vi "fpga_1DAC_sine_and_1ADC_W_risingedge_R_trailingedge_stacked.vi"() -> ()   [LabVIEW 2018]
uses:
  <vilib>/eio/EIONode/EIONode.xnode
  <vilib>/rvi/eio/common/nirviEmuTemplateMethod_errors.vi
panel:
  in  "delay 4 (us)":u32=350
  in  "delay3 (us)":u32=350
  in  "delay 2 (us)":u32=350
  in  "delay 1 (us)":u32=350
  out "ADC4 read":bool[](array[boolean])
  in  "ADC1 write":bool[](array[boolean])=[FALSE, FALSE, FALSE, FALSE, FALSE, TRUE, FALSE, FALSE, FALSE, FALSE, FALSE, FALSE, FALSE, FALSE, FALSE, FALSE]
  out "ADC3 read":bool[](array[boolean])
  in  "ADC4 write":bool[](array[boolean])=[FALSE, FALSE, TRUE, TRUE, FALSE, TRUE, FALSE, FALSE, FALSE, FALSE, FALSE, FALSE, FALSE, FALSE, FALSE, FALSE]
  in  "ADC3 write":bool[](array[boolean])=[FALSE, FALSE, TRUE, FALSE, FALSE, TRUE, FALSE, FALSE, FALSE, FALSE, FALSE, FALSE, FALSE, FALSE, FALSE, FALSE]
  out "ADC2 read":bool[](array[boolean])
  in  "DAC 1 write":bool[](array[boolean])=[FALSE, FALSE, FALSE, FALSE, FALSE, FALSE, FALSE, FALSE, FALSE, FALSE, FALSE, FALSE, FALSE, FALSE, FALSE, FALSE]
  out "ADC1 read":bool[](array[boolean])
  in  "ADC2 write":bool[](array[boolean])=[FALSE, FALSE, FALSE, TRUE, FALSE, TRUE, FALSE, FALSE, FALSE, FALSE, FALSE, FALSE, FALSE, FALSE, FALSE, FALSE]
  in  "delay (us)":u32=350
  in  "Stop":bool
  in  "DAC 2 write":bool[](array[boolean])=[FALSE, FALSE, FALSE, FALSE, FALSE, FALSE, FALSE, FALSE, FALSE, FALSE, FALSE, FALSE, FALSE, FALSE, FALSE, FALSE]
  in  "DAC 3 write":bool[](array[boolean])=[FALSE, FALSE, FALSE, FALSE, FALSE, FALSE, FALSE, FALSE, FALSE, FALSE, FALSE, FALSE, FALSE, FALSE, FALSE, FALSE]
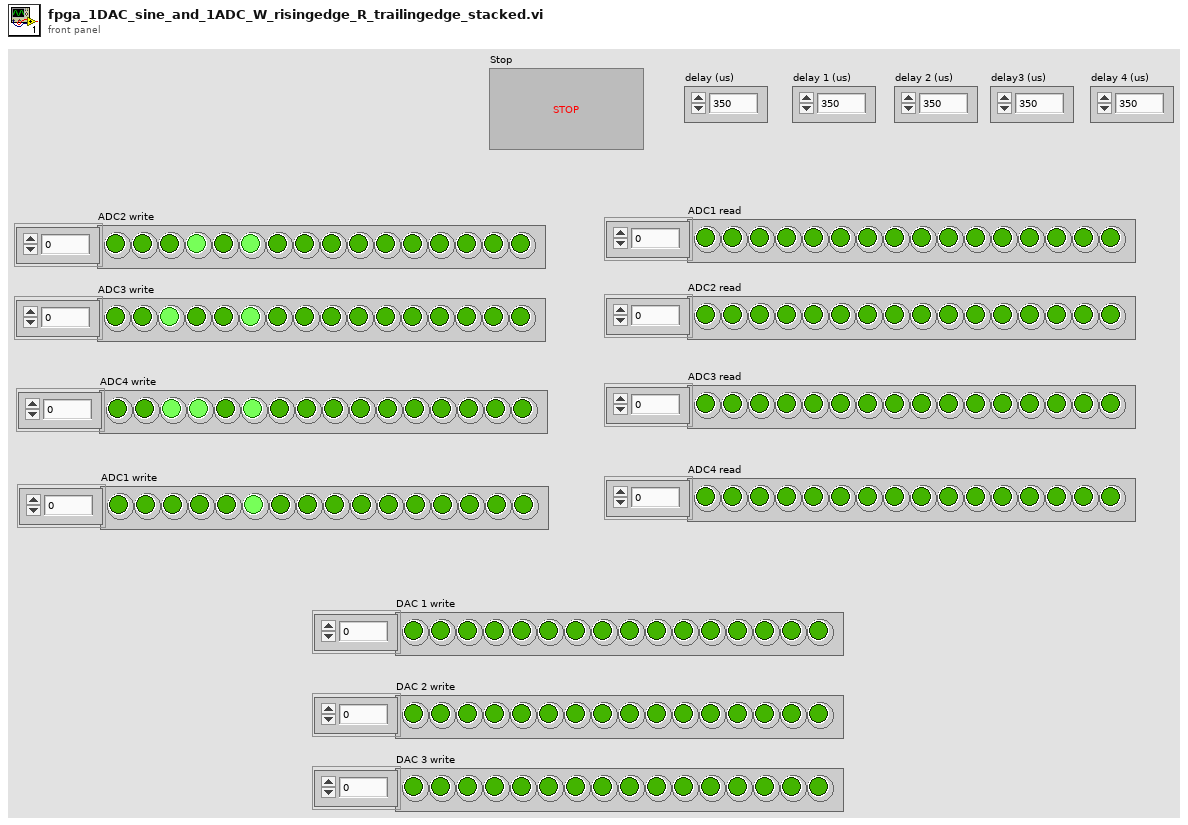
[diagram p1: front panel]
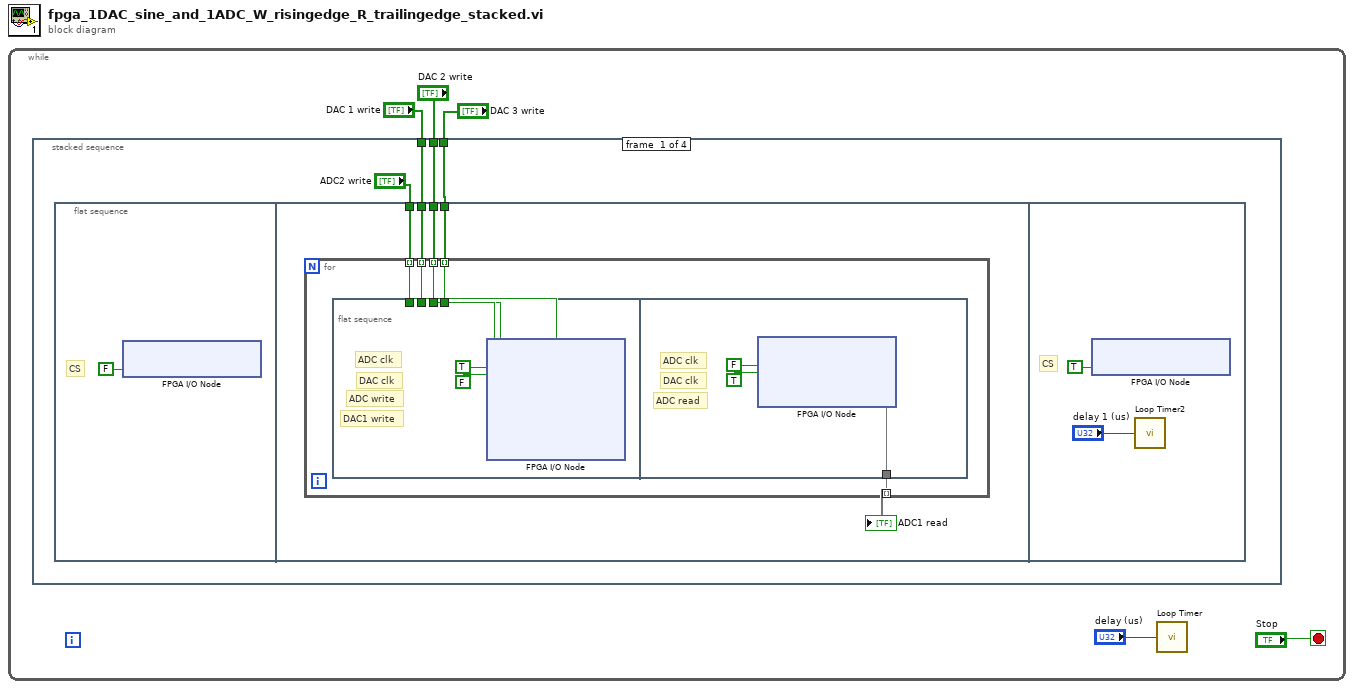
[diagram p0: block diagram]
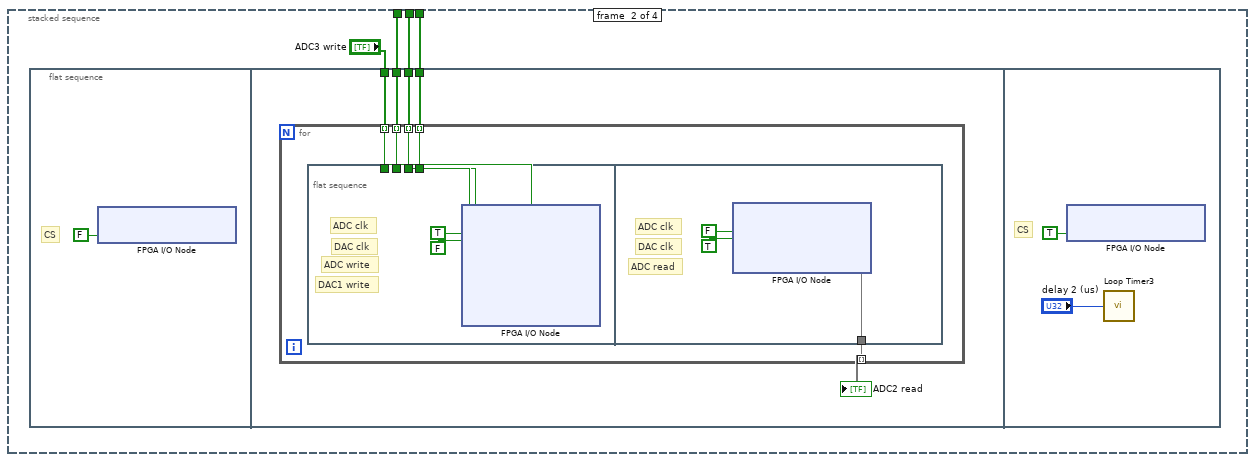
[diagram p2: hidden frame]
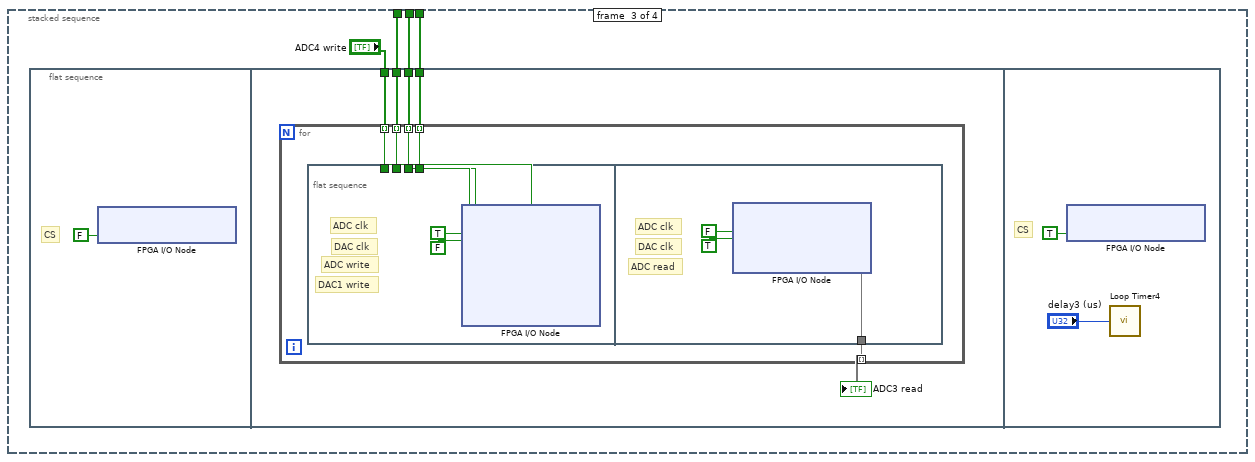
[diagram p3: hidden frame]
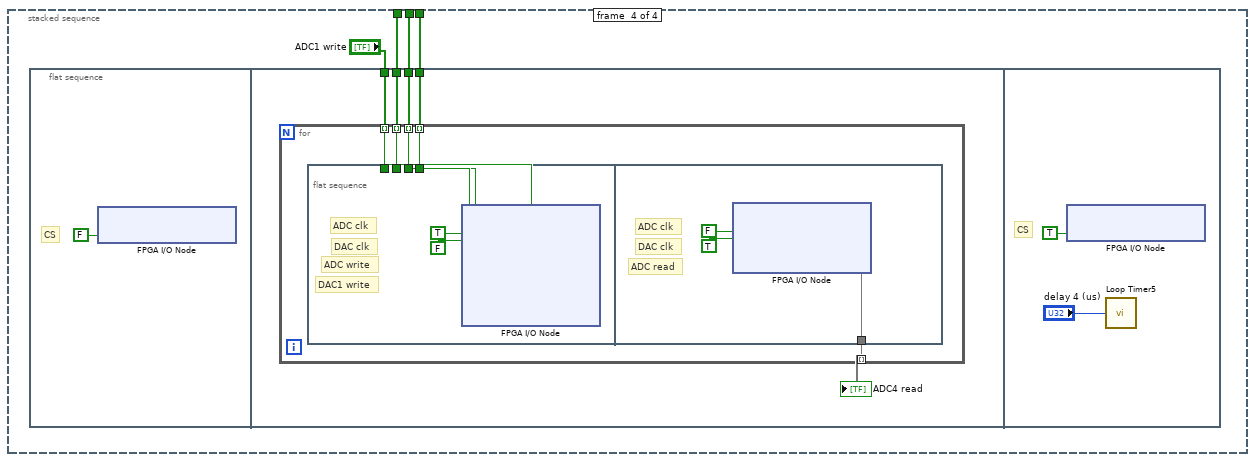
[diagram p4: hidden frame]
diagram:
  n1 = while {
    stop <- "Stop" stop-if-true
    n2 = stacked-sequence {
      tunnel: "DAC 3 write" -> [w8 w32 w58 w84]
      tunnel: "DAC 2 write" -> [w7 w33 w59 w85]
      tunnel: "DAC 1 write" -> [w6 w34 w60 w86]
      frame #0 {
        n3 = flat-sequence {
          tunnel: w6 -> [w15]
          tunnel: "ADC2 write" -> [w14]
          tunnel: w7 -> [w12]
          tunnel: w8 -> [w11]
          frame #0 {
            # "CS"
            n4 = xnode "FPGA I/O Node"("ConnectorA/DIO4"=FALSE) -> ()  [unwired: 1 in, 1 out]
          }
          frame #1 {
            n5 = for {
              tunnel: w15 -> [w20] mode=indexing
              tunnel: w14 -> [w19] mode=indexing
              tunnel: [w18] -> w13 mode=indexing
              tunnel: w12 -> [w17] mode=indexing
              tunnel: w11 -> [w16] mode=indexing
              n6 = flat-sequence {
                tunnel: w20 -> [w23]
                tunnel: w19 -> [w24]
                tunnel: w17 -> [w22]
                tunnel: w16 -> [w21]
                tunnel: [w27] -> w18
                frame #0 {
                  # "DAC1 write"
                  # "ADC write"
                  # "DAC clk"
                  # "ADC clk"
                  n7 = xnode "FPGA I/O Node"("ConnectorA/DIO3"=TRUE, "ConnectorA/DIO5"=FALSE, "ConnectorA/DIO2"=w24, "ConnectorA/DIO6"=w23, "ConnectorA/DIO7"=w22, "ConnectorA/DIO8"=w21) -> ()  [unwired: 6 in, 6 out]
                }
                frame #1 {
                  # "ADC read"
                  # "DAC clk"
                  # "ADC clk"
                  n8 = xnode "FPGA I/O Node"("ConnectorA/DIO3"=FALSE, "ConnectorA/DIO5"=TRUE) -> ("ConnectorA/DIO1"=w27)  [unwired: 3 in, 3 out]
                }
              }
            }
            "ADC1 read" <- w13
          }
          frame #2 {
            # "CS"
            n9 = xnode "FPGA I/O Node"("ConnectorA/DIO4"=TRUE) -> ()  [unwired: 1 in, 1 out]
            n10 = call "Loop Timer2"("Count(Ticks)"="delay 1 (us)") -> ()  [unwired: 1 out]
          }
        }
      }
      frame #1 {
        n11 = flat-sequence {
          tunnel: w34 -> [w41]
          tunnel: "ADC3 write" -> [w40]
          tunnel: w33 -> [w38]
          tunnel: w32 -> [w37]
          frame #0 {
            # "CS"
            n12 = xnode "FPGA I/O Node"("ConnectorA/DIO4"=FALSE) -> ()  [unwired: 1 in, 1 out]
          }
          frame #1 {
            n13 = for {
              tunnel: w41 -> [w46] mode=indexing
              tunnel: w40 -> [w45] mode=indexing
              tunnel: [w44] -> w39 mode=indexing
              tunnel: w38 -> [w43] mode=indexing
              tunnel: w37 -> [w42] mode=indexing
              n14 = flat-sequence {
                tunnel: w46 -> [w49]
                tunnel: w45 -> [w50]
                tunnel: w43 -> [w48]
                tunnel: w42 -> [w47]
                tunnel: [w53] -> w44
                frame #0 {
                  # "DAC1 write"
                  # "ADC write"
                  # "DAC clk"
                  # "ADC clk"
                  n15 = xnode "FPGA I/O Node"("ConnectorA/DIO3"=TRUE, "ConnectorA/DIO5"=FALSE, "ConnectorA/DIO2"=w50, "ConnectorA/DIO6"=w49, "ConnectorA/DIO7"=w48, "ConnectorA/DIO8"=w47) -> ()  [unwired: 6 in, 6 out]
                }
                frame #1 {
                  # "ADC read"
                  # "DAC clk"
                  # "ADC clk"
                  n16 = xnode "FPGA I/O Node"("ConnectorA/DIO3"=FALSE, "ConnectorA/DIO5"=TRUE) -> ("ConnectorA/DIO1"=w53)  [unwired: 3 in, 3 out]
                }
              }
            }
            "ADC2 read" <- w39
          }
          frame #2 {
            # "CS"
            n17 = xnode "FPGA I/O Node"("ConnectorA/DIO4"=TRUE) -> ()  [unwired: 1 in, 1 out]
            n18 = call "Loop Timer3"("Count(Ticks)"="delay 2 (us)") -> ()  [unwired: 1 out]
          }
        }
      }
      frame #2 {
        n19 = flat-sequence {
          tunnel: w60 -> [w67]
          tunnel: "ADC4 write" -> [w66]
          tunnel: w59 -> [w64]
          tunnel: w58 -> [w63]
          frame #0 {
            # "CS"
            n20 = xnode "FPGA I/O Node"("ConnectorA/DIO4"=FALSE) -> ()  [unwired: 1 in, 1 out]
          }
          frame #1 {
            n21 = for {
              tunnel: w67 -> [w72] mode=indexing
              tunnel: w66 -> [w71] mode=indexing
              tunnel: [w70] -> w65 mode=indexing
              tunnel: w64 -> [w69] mode=indexing
              tunnel: w63 -> [w68] mode=indexing
              n22 = flat-sequence {
                tunnel: w72 -> [w75]
                tunnel: w71 -> [w76]
                tunnel: w69 -> [w74]
                tunnel: w68 -> [w73]
                tunnel: [w79] -> w70
                frame #0 {
                  # "DAC1 write"
                  # "ADC write"
                  # "DAC clk"
                  # "ADC clk"
                  n23 = xnode "FPGA I/O Node"("ConnectorA/DIO3"=TRUE, "ConnectorA/DIO5"=FALSE, "ConnectorA/DIO2"=w76, "ConnectorA/DIO6"=w75, "ConnectorA/DIO7"=w74, "ConnectorA/DIO8"=w73) -> ()  [unwired: 6 in, 6 out]
                }
                frame #1 {
                  # "ADC read"
                  # "DAC clk"
                  # "ADC clk"
                  n24 = xnode "FPGA I/O Node"("ConnectorA/DIO3"=FALSE, "ConnectorA/DIO5"=TRUE) -> ("ConnectorA/DIO1"=w79)  [unwired: 3 in, 3 out]
                }
              }
            }
            "ADC3 read" <- w65
          }
          frame #2 {
            # "CS"
            n25 = xnode "FPGA I/O Node"("ConnectorA/DIO4"=TRUE) -> ()  [unwired: 1 in, 1 out]
            n26 = call "Loop Timer4"("Count(Ticks)"="delay3 (us)") -> ()  [unwired: 1 out]
          }
        }
      }
      frame #3 {
        n27 = flat-sequence {
          tunnel: w86 -> [w93]
          tunnel: "ADC1 write" -> [w92]
          tunnel: w85 -> [w90]
          tunnel: w84 -> [w89]
          frame #0 {
            # "CS"
            n28 = xnode "FPGA I/O Node"("ConnectorA/DIO4"=FALSE) -> ()  [unwired: 1 in, 1 out]
          }
          frame #1 {
            n29 = for {
              tunnel: w93 -> [w98] mode=indexing
              tunnel: w92 -> [w97] mode=indexing
              tunnel: [w96] -> w91 mode=indexing
              tunnel: w90 -> [w95] mode=indexing
              tunnel: w89 -> [w94] mode=indexing
              n30 = flat-sequence {
                tunnel: w98 -> [w101]
                tunnel: w97 -> [w102]
                tunnel: w95 -> [w100]
                tunnel: w94 -> [w99]
                tunnel: [w105] -> w96
                frame #0 {
                  # "DAC1 write"
                  # "ADC write"
                  # "DAC clk"
                  # "ADC clk"
                  n31 = xnode "FPGA I/O Node"("ConnectorA/DIO3"=TRUE, "ConnectorA/DIO5"=FALSE, "ConnectorA/DIO2"=w102, "ConnectorA/DIO6"=w101, "ConnectorA/DIO7"=w100, "ConnectorA/DIO8"=w99) -> ()  [unwired: 6 in, 6 out]
                }
                frame #1 {
                  # "ADC read"
                  # "DAC clk"
                  # "ADC clk"
                  n32 = xnode "FPGA I/O Node"("ConnectorA/DIO3"=FALSE, "ConnectorA/DIO5"=TRUE) -> ("ConnectorA/DIO1"=w105)  [unwired: 3 in, 3 out]
                }
              }
            }
            "ADC4 read" <- w91
          }
          frame #2 {
            # "CS"
            n33 = xnode "FPGA I/O Node"("ConnectorA/DIO4"=TRUE) -> ()  [unwired: 1 in, 1 out]
            n34 = call "Loop Timer5"("Count(Ticks)"="delay 4 (us)") -> ()  [unwired: 1 out]
          }
        }
      }
    }
    n35 = call "Loop Timer"("Count(Ticks)"="delay (us)") -> ()  [unwired: 1 out]
  }
